vi "SMC_INIT.vi"(8 "error in (no error)":errorcluster, 10 "SMC Parameter":T1={"VENUS Language"=enum."VENUS 2", "Number of Axis"=4, "Controller Nr"=3, "Simulation"=FALSE} {"Controller Nr" min=1 max=10 step=1}, 11 "Communication Parameter":T3={"Comm Method"=enum."RS232", "Com Port"=1, "Baud Rate"=9600, "IP Address"="10.0.10.84", "Remote Port"=23, "GPIB Address"="", "VISA Resource Name"="", "Visa Baud Rate"=9600, "Visa Serial"=FALSE}) -> (0 "error out":errorcluster)   [LabVIEW 2015]
uses:
  SubVIs/JS_Comm.llb/Comm_Paras.ctl
  SubVIs/JS_Comm.llb/Comm_Method.ctl
  SMC_SubVIs.llb/SMC Paras.ctl
  SMC_SubVIs.llb/VENUSNr.ctl
  SMC_SubVIs.llb/SMC_ManagerMode.ctl
  SubVIs/JS_Comm.llb/Communication_Job.ctl
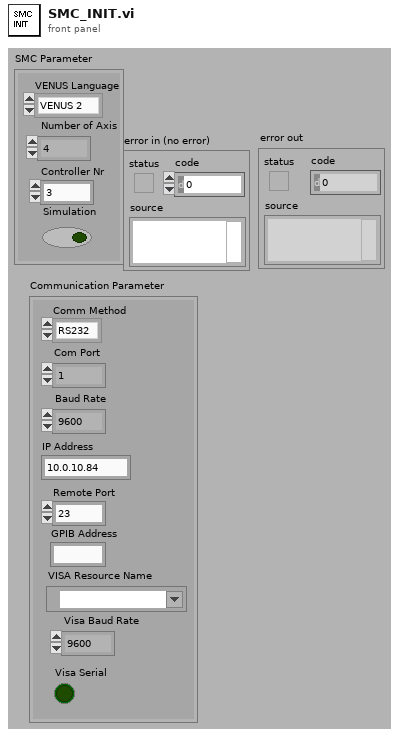
[diagram p1: front panel]
types:
  T1 = typedef "SMC Paras.ctl" = cluster{"VENUS Language":T2, "Number of Axis":u8, "Controller Nr":u8, "Simulation":bool}
  T2 = typedef "VENUSNr.ctl" = enum16{"VENUS 2", "VENUS 1"}
  T3 = typedef "Comm_Paras.ctl" = cluster{"Comm Method":T4, "Com Port":i32, "Baud Rate":u32, "IP Address":string, "Remote Port":u16, "GPIB Address":string, "VISA Resource Name":refnum<visa-resource-name>, "Visa Baud Rate":u32, "Visa Serial":bool}
  T4 = typedef "Comm_Method.ctl" = enum16{"RS232", "TCPIP", "GPIB", "VISA"}
  T5 = typedef "Communication_Job.ctl" = enum16{"Init", "Read", "hasLF", "Get1Line", "Write", "Close", "Clear"}
  T6 = typedef "SMC_ManagerMode.ctl" = enum16{"Init", "Get", "SetPosition", "SetStatus", "SetMoving", "SetControllerNr"}
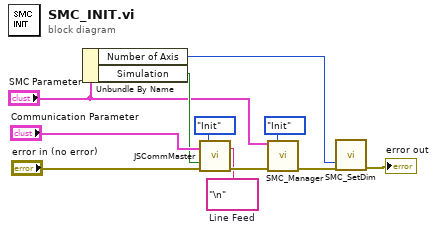
[diagram p0: block diagram]
diagram:
  w1 = "\n"  # Line Feed
  n1 = Unbundle By Name("SMC Parameter") -> ("Number of Axis"=w2:u8, "Simulation"=w4:bool)
  n2 = call "JSCommMaster.vi"("CommJob"=Communication_Job."Init", "Communication Parameter"="Communication Parameter", "termCharRead"=w1, "Simulation"=w4, "error in (no error)"="error in (no error)") -> ("error out"=w8:errorcluster)  [unwired: 8 in, 2 out]
  n3 = call "SMC_Manager.vi"("SMC Parameter"="SMC Parameter", "Mode"=SMC_ManagerMode."Init", "error in (no error)"=w8) -> ("error out"=w10:errorcluster)  [unwired: 8 in, 4 out]
  n4 = call "SMC_SetDim.vi"("error in (no error)"=w10, "Dimension"=w2) -> ("error out"=→"error out":errorcluster)  [unwired: 9 in]
